vi "plot_update_cursorPos_sub.vi"(0 "min":sgl format="%.2f", 2 "max":sgl format="%.2f", 4 "factor":sgl format="%.2f") -> (14 "min":sgl format="%.2f", 16 "max":sgl format="%.2f")   [LabVIEW 2010, in "OSA.lvclass"]
doc: "SubVI to a <B>Thorlabs_OSA_64</B> object.\n\n[GOOP 1.0]"
uses:
  OSA.lvclass
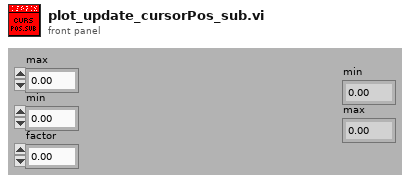
[diagram p1: front panel]
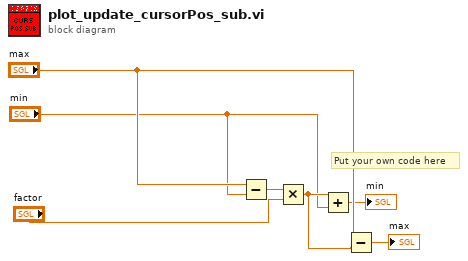
[diagram p0: block diagram]
diagram:
  # "Put your own code here"
  n1 = Subtract(x="max", y="min") -> (x-y=w7:sgl)
  n2 = Multiply(x=w7, y="factor") -> (x*y=w6:sgl)
  n3 = Add(x=w6, y="min") -> (x+y=→"min":sgl)
  n4 = Subtract(x="max", y=w6) -> (x-y=→"max":sgl)
